vi "ModifyImage ctab.vi"(8 "error in (no error)":errorcluster, 11 "ITX Commands in":refnum<class "ITX Commands.lvclass">) -> (0 "error out":errorcluster, 3 "ITX Commands out":refnum<class "ITX Commands.lvclass">)   [LabVIEW 2016, in "ITX Commands.lvclass"]
uses:
  ITX Commands.lvclass
panel:
  out "resulting string":string
  in  "Invert Color Scheme?":bool
  in  "Color Table Name":string
  # "Some Example Color Table Names \n(More on pg. 401 of Igor manual):"
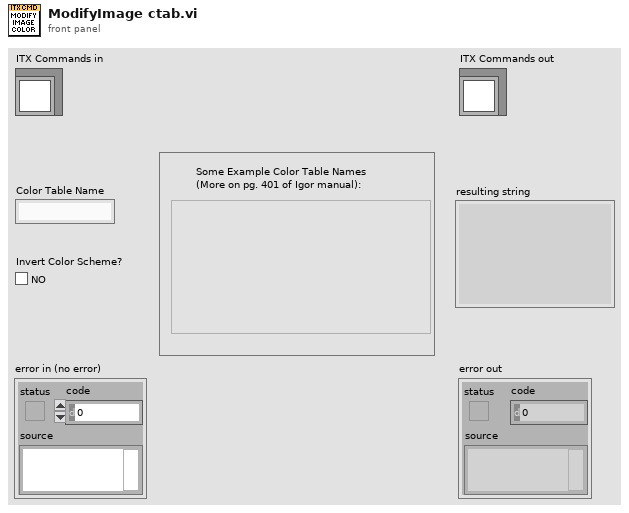
[diagram p1: front panel]
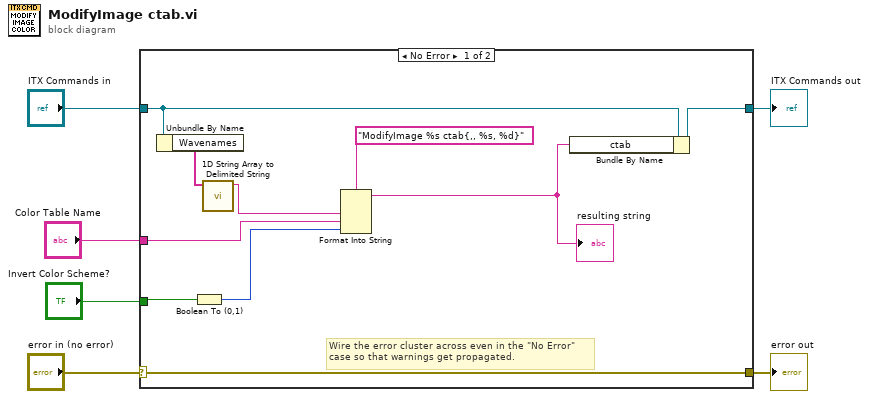
[diagram p0: block diagram]
diagram:
  n1 = case shown="No Error" "error in (no error)" {
    selector: "error in (no error)" -> [w16 w18]
    tunnel: [w16 w18] -> w5
    tunnel: [w13 w17] -> w3
    tunnel: "ITX Commands in" -> [w11 w17]
    tunnel: "Color Table Name" -> [w8 _]
    tunnel: "Invert Color Scheme?" -> [w14 _]
    frame No Error {
      # "Wire the error cluster across even in the \"No Error\"\ncase so that warnings get propagated."
      n2 = Unbundle By Name(w11) -> ("Wavenames"=w10:string[])
      n3 = Boolean To (0,1)(Boolean=w14) -> (0, 1=w7:i16)
      n4 = call <vilib>:"1D String Array to Delimited String.vi"("string array"=w10) -> ("delimited string"=w9:string)  [unwired: 10 in]
      n5 = Format Into String(format string="ModifyImage %s ctab{,, %s, %d}", w9, w8, w7) -> (resulting string=w12:string)  [unwired: 2 in, 1 out]
      "resulting string" <- w12
      n6 = Bundle By Name(cluster=w11, "ctab"=w12) -> (w13:refnum<class "ITX Commands.lvclass">)
    }
    frame Error {
    }
  }
  "error out" <- w5
  "ITX Commands out" <- w3
